vi "LEO TESTA MINCHIATA.vi"() -> ()   [LabVIEW 2014]
panel:
  out "size signal":i32
  out "size FFT":i32
  out "FFT Chart":i16[](graph)
  out "Signal Chart":i16[](graph)
  in  "Snapshot-UI":bool
  in  "snapshot-FPGA":bool
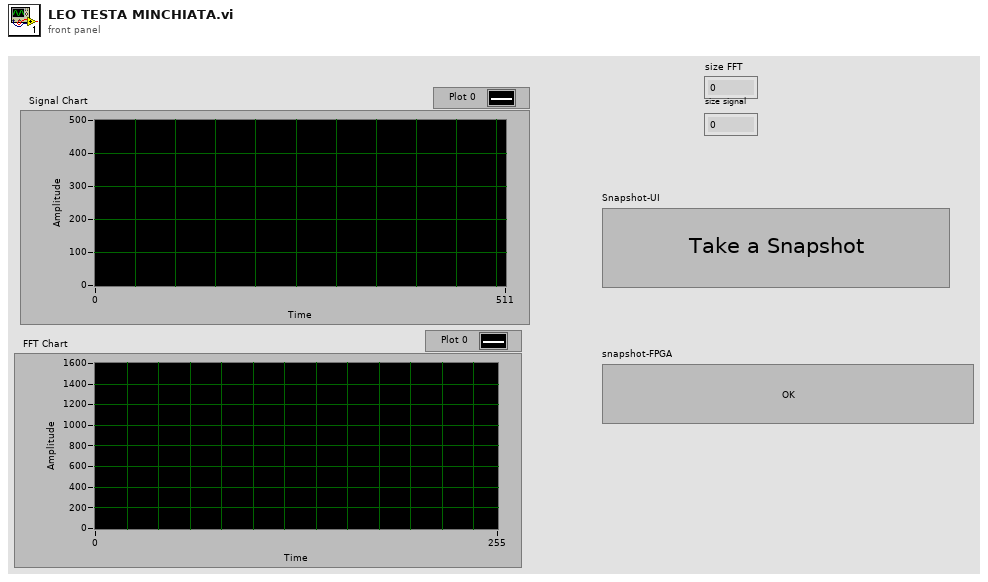
[diagram p1: front panel]
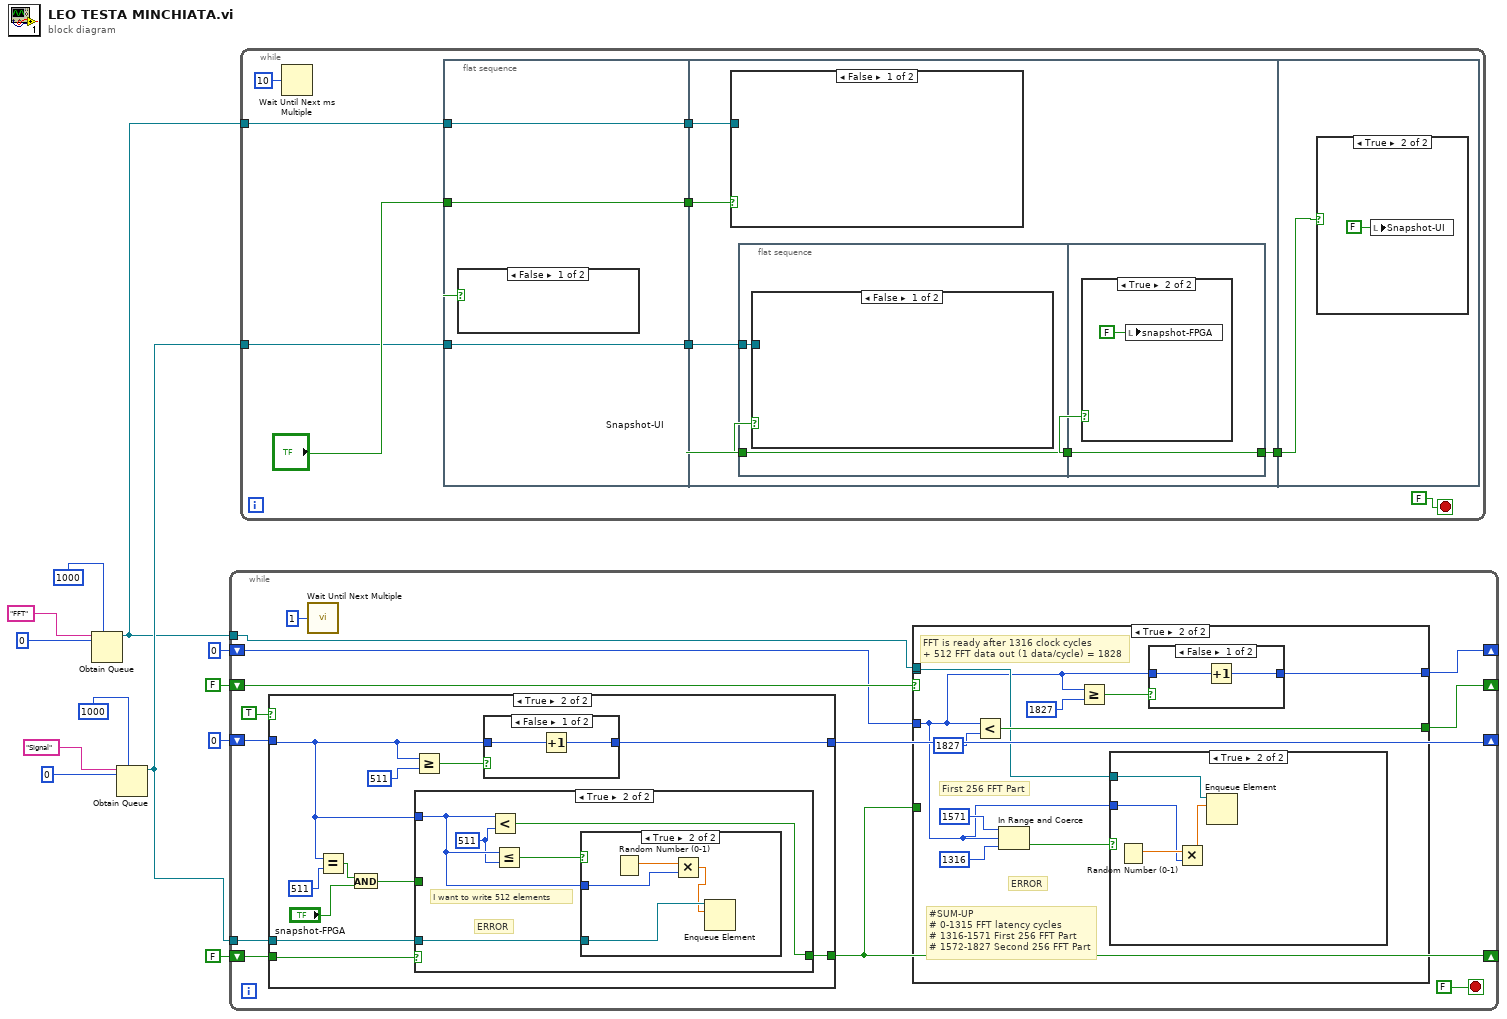
[diagram p0: block diagram]
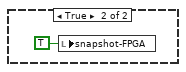
[diagram p2: hidden frame]
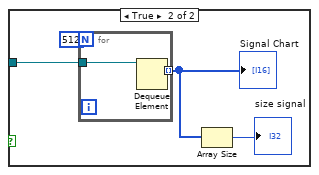
[diagram p3: hidden frame]
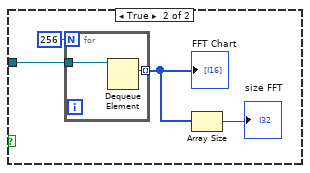
[diagram p5: hidden frame]
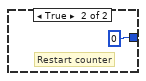
[diagram p9: hidden frame]
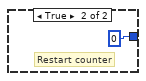
[diagram p13: hidden frame]
diagram:
  n1 = Obtain Queue(max queue size (-1, unlimited)=1000, name (unnamed)="FFT", element data type=i16 0) -> (queue out=w1:refnum<queue>)  [unwired: 2 in, 2 out]
  n2 = Obtain Queue(max queue size (-1, unlimited)=1000, name (unnamed)="Signal", element data type=i16 0) -> (queue out=w2:refnum<queue>)  [unwired: 2 in, 2 out]
  n3 = while {
    shift-right: [w22] -> _
    shift-left: FALSE -> [w24]
    shift-right: [w25] -> _
    shift-left: i16 0 -> [w23]
    shift-right: [w21] -> _
    shift-left: FALSE -> [w20]
    shift-right: [w18] -> _
    shift-left: i16 0 -> [w19]
    tunnel: w2 -> [w17]
    tunnel: w1 -> [w16]
    stop <- FALSE stop-if-true
    n4 = case shown="True" TRUE {
      tunnel: w23 -> [w46 w50]
      tunnel: [w46 w55] -> w25
      tunnel: w24 -> [w45 w48]
      tunnel: [w45 w49] -> w22
      tunnel: w17 -> [_ w47]
      frame False {
      }
      frame True {
        n5 = Equal?(x=w50, y=i16 511) -> (x = y?=w54:bool)
        n6 = And(x=w54, y="snapshot-FPGA") -> (x .and. y?=w51:bool)
        n7 = Greater Or Equal?(x=w50, y=i16 511) -> (x >= y?=w56:bool)
        n8 = case shown="True" w48 {
          tunnel: w51 -> [w58 _]
          tunnel: w50 -> [_ w60]
          tunnel: [w58 w63] -> w49
          tunnel: w47 -> [_ w61]
          frame False {
          }
          frame True {
            w59 = i16 511 ("y")
            # "ERROR"
            # "I want to write 512 elements"
            n9 = Less?(x=w60, y=w59) -> (x < y?=w63:bool)
            n10 = Less Or Equal?(x=w60, y=w59) -> (x <= y?=w62:bool)
            n11 = case shown="True" w62 {
              tunnel: w61 -> [_ w67]
              tunnel: w60 -> [_ w66]
              frame False {
              }
              frame True {
                n12 = Random Number (0-1)() -> (number: 0 to 1=w64:dbl)
                n13 = Multiply(x=w64, y=w66) -> (x*y=w65:dbl)
                n14 = Enqueue Element(queue=w67, element=w65) -> ()  [unwired: 2 in, 3 out]
              }
            }
          }
        }
        n15 = case shown="False" w56 {
          tunnel: w50 -> [w69 _]
          tunnel: [w68 i16 0] -> w55
          frame False {
            n16 = Increment(x=w69) -> (x+1=w68:i16)
          }
          frame True {
            # "Restart counter"
          }
        }
      }
    }
    n17 = call "Wait Until Next Multiple"("Count(mSec)"=u32 1) -> ()  [unwired: 1 out]
    n18 = case shown="True" w20 {
      tunnel: w22 -> [w27 _]
      tunnel: [w27 w37] -> w21
      tunnel: w19 -> [w26 w28]
      tunnel: [w26 w33] -> w18
      tunnel: [_ w29] -> _
      tunnel: w16 -> [_ w29]
      frame False {
      }
      frame True {
        # "ERROR"
        # "First 256 FFT Part"
        # "#SUM-UP\n# 0-1315 FFT latency cycles\n# 1316-1571 First 256 FFT Part\n# 1572-1827 Second 256 FFT Part"
        # "FFT is ready after 1316 clock cycles\n+ 512 FFT data out (1 data/cycle) = 1828"
        n19 = Less?(x=w28, y=i16 1827) -> (x < y?=w37:bool)
        n20 = In Range and Coerce(upper limit=i16 1571, x=w28, lower limit=i16 1316 ("y")) -> (In Range?=w30:bool)  [unwired: 1 out]
        n21 = Greater Or Equal?(x=w28, y=i16 1827) -> (x >= y?=w34:bool)
        n22 = case shown="True" w30 {
          tunnel: w29 -> [_ w41]
          tunnel: w28 -> [_ w39]
          frame False {
          }
          frame True {
            n23 = Random Number (0-1)() -> (number: 0 to 1=w40:dbl)
            n24 = Multiply(x=w40, y=w39) -> (x*y=w38:dbl)
            n25 = Enqueue Element(queue=w41, element=w38) -> ()  [unwired: 2 in, 3 out]
          }
        }
        n26 = case shown="False" w34 {
          tunnel: w28 -> [w43 _]
          tunnel: [w42 i16 0] -> w33
          frame False {
            n27 = Increment(x=w43) -> (x+1=w42:i16)
          }
          frame True {
            # "Restart counter"
          }
        }
      }
    }
  }
  n28 = while {
    tunnel: w2 -> [w78]
    tunnel: w1 -> [w77]
    stop <- FALSE stop-if-true
    n29 = Wait Until Next ms Multiple(millisecond multiple=u32 10) -> ()  [unwired: 1 out]
    n30 = flat-sequence {
      tunnel: w77 -> [w81]
      tunnel: w78 -> [w82]
      tunnel: "Snapshot-UI" -> [w80]
      tunnel: [w80] -> w75
      tunnel: [w82] -> w74
      tunnel: [w81] -> w73
      tunnel: w75 -> [w87]
      tunnel: w74 -> [w86]
      tunnel: w73 -> [w85]
      tunnel: [w84] -> w71
      tunnel: w71 -> [w105]
      frame #0 {
        n31 = case shown="False" w80 {
          frame False {
          }
          frame True {
            n32 = local write "snapshot-FPGA"(TRUE ("snapshot-FPGA")) -> ()
          }
        }
      }
      frame #1 {
        n33 = case shown="False" w87 {
          tunnel: w85 -> [_ w101]
          frame False {
          }
          frame True {
            n34 = for {
              N: 256 -> [_]
              tunnel: [w104] -> w100 mode=indexing
              tunnel: w101 -> [w103]
              n35 = Dequeue Element(queue=w103) -> (element=w104:i16)  [unwired: 2 in, 3 out]
            }
            "FFT Chart" <- w100
            n36 = Array Size(array=w100) -> (size(s)=→"size FFT":i32)
          }
        }
        n37 = flat-sequence {
          tunnel: w87 -> [w90]
          tunnel: [w90] -> w88
          tunnel: w86 -> [w89]
          tunnel: w88 -> [w97]
          tunnel: [w97] -> w84
          frame #0 {
            n38 = case shown="False" w90 {
              tunnel: w89 -> [_ w94]
              frame False {
              }
              frame True {
                n39 = for {
                  N: 512 -> [_]
                  tunnel: w94 -> [w96]
                  tunnel: [w95] -> w91 mode=indexing
                  n40 = Dequeue Element(queue=w96) -> (element=w95:i16)  [unwired: 2 in, 3 out]
                }
                "Signal Chart" <- w91
                n41 = Array Size(array=w91) -> (size(s)=→"size signal":i32)
              }
            }
          }
          frame #1 {
            n42 = case shown="True" w97 {
              frame False {
              }
              frame True {
                n43 = local write "snapshot-FPGA"(FALSE ("snapshot")) -> ()
              }
            }
          }
        }
      }
      frame #2 {
        n44 = case shown="True" w105 {
          frame False {
          }
          frame True {
            n45 = local write "Snapshot-UI"(FALSE ("Snapshot-UI")) -> ()
          }
        }
      }
    }
  }
